vi "HeaderAction.vi"(0 "InstrClass":refnum<class "SR400.lvclass"> caption="DNL_LabVIEW Object in", 11 "error in (no error)":errorcluster caption="entrée d'erreur (pas d'erreur)") -> (4 "InstrClassOut":refnum<class "SR400.lvclass"> caption="DNL_LabVIEW Object out", 6 "DataNames":string[](array[string]), 8 "Instr Name":string, 10 "HeaderString":string, 13 "ArrDisplayNames":string[](array[string]), 14 "DisplayNames":string[](array[string]), 15 "error out":errorcluster caption="sortie d'erreur")   [LabVIEW 2019, in "SR400.lvclass"]
uses:
  SR400.lvclass
  C:/Programmes Labview/LabScanV1A/DevicesClass/BaseDevice/BaseDevice.lvclass
  SR400.lvclass/SR400.ctl
  BaseDevice/BaseDevice.lvclass
panel:
  in  "Mode":u16(ring) items=["A,B for T Preset", "A-B for T Preset", "A+B for T Preset", "A for B preset"]
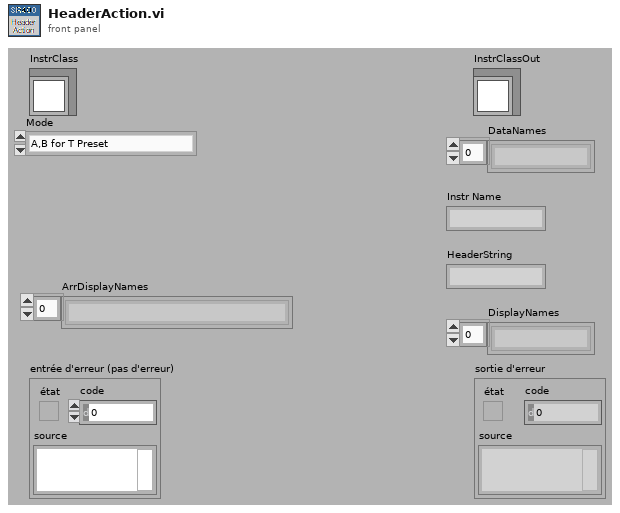
[diagram p1: front panel]
types:
  T1 = typedef "SR400.lvclass/SR400_Func.ctl" = enum16{"Read_Count (Arb)"}
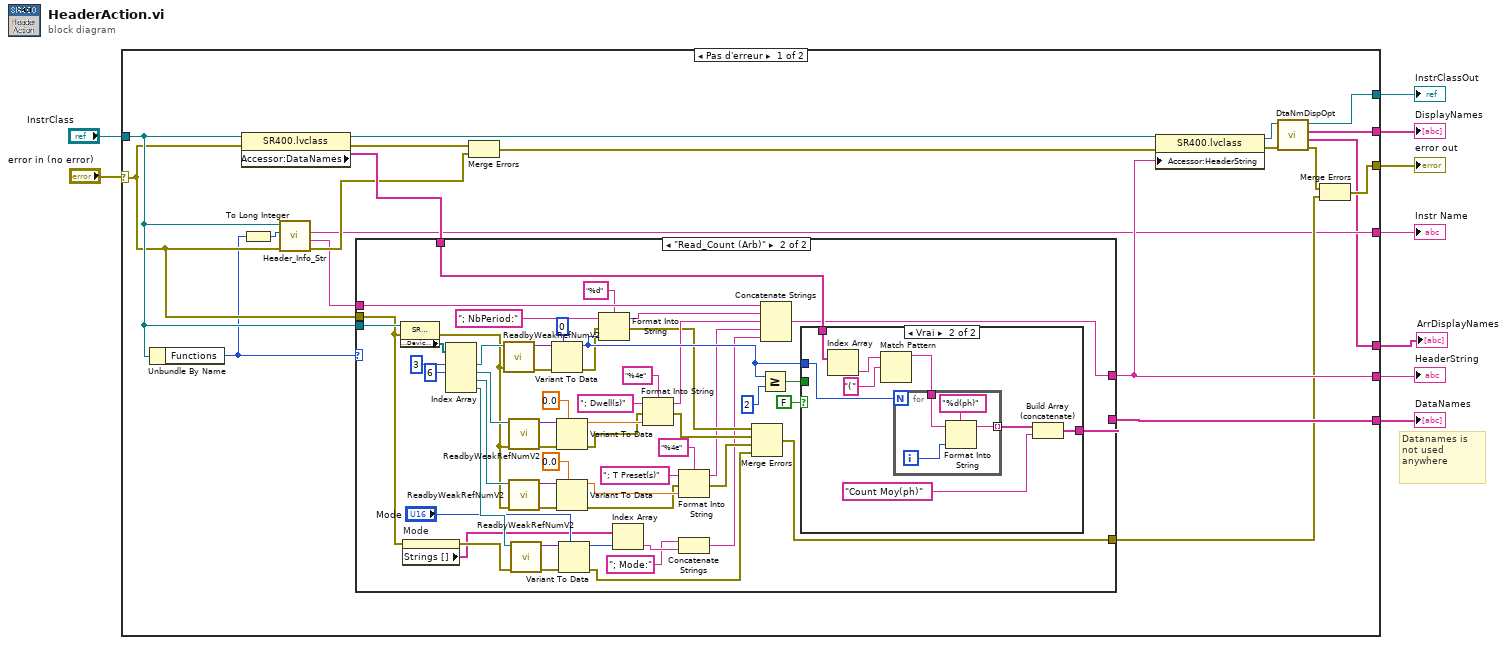
[diagram p0: block diagram]
diagram:
  # "Datanames is not used anywhere"
  n1 = case shown="Pas d'erreur" "error in (no error)" {
    selector: "error in (no error)" -> [w15 w102]
    tunnel: [w28 _] -> w8
    tunnel: [w21 _] -> w7
    tunnel: "InstrClass" -> [w17 w103]
    tunnel: [w18 w102] -> w5
    tunnel: [w26 w103] -> w3
    tunnel: [w13 _] -> w4
    tunnel: [w24 _] -> w2
    tunnel: [w10 _] -> w1
    frame No Error {
      n2 = Unbundle By Name(w17) -> ("Functions"=w11:T1)
      n3 = property class="SR400.lvclass"(reference=w17, error in=w15) -> (reference out=w30:refnum<class "SR400.lvclass">, error out=w29:errorcluster, "Accessor:DataNames"=w22:string[])
      n4 = To Long Integer(number=w11) -> (32bit integer=w12:i32)
      n5 = call-dynamic "Header_Info_Str.vi"("error in (no error)"=w15, "Functions"=w12, "DefaultDev in"=w17) -> ("error out"=w16:errorcluster, "HdrInfoStr"=w14:string, "InstrumentName"=w13:string)  [unwired: 5 in, 1 out]
      n6 = case shown="\"Read_Count (Arb)\"" w11 {
        tunnel: [w33 w34] -> w28
        tunnel: w14 -> [w33 w86]
        tunnel: w22 -> [w32 w82]
        tunnel: w17 -> [_ w87]
        tunnel: w15 -> [w31 w54]
        tunnel: [w32 w76] -> w21
        tunnel: [w31 w37] -> w19
        frame Default {
        }
        frame "Read_Count (Arb)" {
          n7 = property class="SR400.lvclass"(reference=w87, error in=w54) -> (error out=w53:errorcluster, "Accessor:DeviceCtrl"=w65:refnum<vi>[])  [unwired: 1 out]
          n8 = property on="Mode" class="MDér (strict)"(error in=w54) -> (error out=w52:errorcluster, "Strings []"=w51:string[])  [unwired: 1 in, 1 out]
          n9 = Index Array(array=w65, index #1=3 ("index"), index #2=6 ("index")) -> (element #1=w84:refnum<vi>, element #2=w72:refnum<vi>, element #3=w68:refnum<vi>, element #4=w66:refnum<vi>)  [unwired: 2 in]
          n10 = call <userlib>:"ReadbyWeakRefNumV2.vi"("error in"=w53, "Control Ref"=w84) -> ("error out"=w59:errorcluster, "Valeur"=w88:variant)  [unwired: 8 in]
          n11 = call <userlib>:"ReadbyWeakRefNumV2.vi"("error in"=w53, "Control Ref"=w72) -> ("error out"=w60:errorcluster, "Valeur"=w71:variant)  [unwired: 8 in]
          n12 = call <userlib>:"ReadbyWeakRefNumV2.vi"("error in"=w53, "Control Ref"=w68) -> ("error out"=w62:errorcluster, "Valeur"=w69:variant)  [unwired: 8 in]
          n13 = call <userlib>:"ReadbyWeakRefNumV2.vi"("error in"=w52, "Control Ref"=w66) -> ("error out"=w61:errorcluster, "Valeur"=w63:variant)  [unwired: 8 in]
          n14 = Variant To Data(error in=w59, type=0 ("Nb de période"), Variant=w88) -> (data=w79:i32, error out=w42:errorcluster)
          n15 = Variant To Data(error in=w60, type=0.0, Variant=w71) -> (data=w48:dbl, error out=w46:errorcluster)
          n16 = Variant To Data(error in=w62, type=0.0, Variant=w69) -> (data=w44:dbl, error out=w43:errorcluster)
          n17 = Variant To Data(error in=w61, type="Mode", Variant=w63) -> (data=w55:u16, error out=w38:errorcluster)
          n18 = Format Into String(format string="%d", initial string="; NbPeriod:", error in=w42, w79) -> (resulting string=w77:string, error out=w41:errorcluster)
          n19 = Index Array(array=w51, index=w55) -> (element=w50:string)
          n20 = Format Into String(format string="%4e", initial string="; Dwell(s)", error in=w46, w48) -> (resulting string=w45:string, error out=w40:errorcluster)
          n21 = Format Into String(format string="%4e", initial string="; T Preset(s)", error in=w43, w44) -> (resulting string=w36:string, error out=w39:errorcluster)
          n22 = Concatenate Strings("; Mode:" ("initial string"), w50) -> (w35:string)
          n23 = Merge Errors(w41, w40, w39, w38) -> (w37:errorcluster)
          n24 = Greater Or Equal?(x=w79, y=2) -> (x >= y?=w75:bool)
          n25 = Concatenate Strings(w86, w77, w45, w36, w35) -> (w34:string)
          n26 = case shown="Vrai" FALSE {
            tunnel: w82 -> [w89 w97]
            tunnel: w79 -> [_ w95]
            tunnel: [w89 w94] -> w76
            tunnel: w75 -> [_ _]
            frame False {
            }
            frame True {
              n27 = Index Array(array=w97) -> (element=w90:string)  [unwired: 1 in]
              n28 = Match Pattern(string=w90, regular expression="(") -> (before substring=w91:string)  [unwired: 1 in, 3 out]
              n29 = for {
                N: w95 -> [_]
                tunnel: w91 -> [w98]
                tunnel: [w99] -> w96 mode=indexing
                i -> [w100]
                n30 = Format Into String(format string="%d(ph)", initial string=w98, w100) -> (resulting string=w99:string)  [unwired: 1 in, 1 out]
              }
              n31 = Build Array (concatenate)(w96, "Count Moy(ph)" ("initial string")) -> (w94:string[])
            }
          }
        }
      }
      n32 = Merge Errors(w29, w16) -> (w23:errorcluster)
      n33 = property class="SR400.lvclass"(reference=w30, error in=w23, "Accessor:HeaderString"=w28) -> (reference out=w25:refnum<class "SR400.lvclass">, error out=w27:errorcluster)
      n34 = call "DtaNmDispOpt.vi"("error in (no error)"=w27, "BaseDevice en entrée"=w25) -> ("error out"=w20:errorcluster, "ArrDisplayNames"=w10:string[], "DisplayNames"=w24:string[], "BaseDevice en sortie"=w26:refnum<class "SR400.lvclass">)  [unwired: 6 in]
      n35 = Merge Errors(w20, w19) -> (w18:errorcluster)
    }
    frame Error {
    }
  }
  "error out" <- w5
  "InstrClassOut" <- w3
  "DataNames" <- w7
  "HeaderString" <- w8
  "Instr Name" <- w4
  "DisplayNames" <- w2
  "ArrDisplayNames" <- w1
